vi "Dashboard Main.vi"() -> ()   [LabVIEW 2018]
uses:
  <vilib>/Utility/miscctls.llb/LVRowAndColumnTypeDef.ctl
  <vilib>/event_ctls.llb/eventvkey.ctl
  <vilib>/Rock Robotics/Network Tables/NT Read Numeric Array.vi
  <vilib>/Rock Robotics/WPI/Dashboard/WPI_DashboardLogging Global.vi
  <vilib>/Utility/inputDevices.llb/keyboardAcquire.vi
panel:
  out "keys pressed":T1(ring)=enum."RIGHT"
  in  "Camera Settings Right":T2={"Frame Rate"=30, "Compression"=30, "Size"=1, "DB Camera Config"=FALSE} {"Frame Rate" scale=1.0..30.0; "Compression" scale=100.0..-1.0; "Size" items=["640x480", "320x240", "160x120"]}
  in  "Camera Name Right":string(combo)="No Camera Selection"
  out "Camera Perf":string
  in  "Camera Settings":T2={"Frame Rate"=30, "Compression"=30, "Size"=1, "DB Camera Config"=FALSE} {"Frame Rate" scale=1.0..30.0; "Compression" scale=100.0..-1.0; "Size" items=["640x480", "320x240", "160x120"]}
  in  "TCP":refnum<k5>
  in  "Rec Mode":enum32{"Stop", "Record", "Playback"}(radio)
  out "Robot IP":string
  out "Image Message":string="Timeout in Camera Communications"
  in  "Dashboard Tab":T3(tab)
  out "tour hauteur":dbl(slide) caption="Slide 2" scale=0.0..500.0
  out "Encodeur tour":dbl(slide) caption="Slide" scale=0.0..500.0
  in  "Select Auto":string(combo)="Select Autonomous ..."
  out "NT Connection":bool
  out "MotorChart R":cluster{"Numeric":dbl, "Numeric":dbl}(graph)
  out "MotorChart L":cluster{"Numeric":dbl, "Numeric":dbl}(graph)
  out "MotorSliders R":cluster{"MotorSlide1":dbl, "MotorSlide2":dbl} {"MotorSlide2" scale=-1.0..1.0 scale format="%#_2e"; "MotorSlide1" scale=-1.0..1.0 scale format="%#_2e"}
  out "MotorSliders L":cluster{"MotorSlide1":dbl, "MotorSlide2":dbl} {"MotorSlide2" scale=-1.0..1.0 scale format="%#_2e"; "MotorSlide1" scale=-1.0..1.0 scale format="%#_2e"}
  out "JS1 Z":dbl(slide) scale=-1.0..1.0 scale format="%#_2e"
  out "JS1 Graph":cluster{"X":dbl, "Y":dbl}[](graph)
  out "JS1 Buttons":T4
  out "JS2 Z":dbl(slide) scale=-1.0..1.0 scale format="%#_2e"
  out "JS2 Graph":cluster{"X":dbl, "Y":dbl}[](graph)
  out "JS2 Buttons":T4
  out "Mode":T5(ring)=enum."Auto Disabled"
  out "Right Camera Perf":cluster{"Bandwidth (Mbps)":dbl, "FPS":dbl}
  out "Camera Image Right":T6(plugin-control)
  in  "DB/String 9":string
  in  "DB/String 8":string
  in  "DB/String 7":string
  in  "DB/String 6":string
  in  "DB/String 5":string
  in  "DB/String 4":string
  in  "DB/String 3":string
  in  "DB/String 2":string
  in  "DB/String 1":string
  in  "DB/String 0":string
  in  "DB/Slider 0":dbl(slide) scale=0.0..5.0
  in  "DB/Slider 1":dbl(slide) scale=0.0..5.0
  in  "DB/Slider 2":dbl(slide) scale=0.0..5.0
  in  "DB/Slider 3":dbl(slide) scale=0.0..5.0
  out "DB/LED 3":bool
  out "DB/LED 2":bool
  out "DB/LED 1":bool
  out "DB/LED 0":bool
  in  "DB/Button 3":bool
  in  "DB/Button 2":bool
  in  "DB/Button 1":bool
  in  "DB/Button 0":bool caption="New Name"
  in  "Test Slider":dbl(slide) scale=0.0..100.0 scale format="%#_3g"
  in  "On/Off":bool caption="Solenoid"
  in  "Test Name":u16(ring) items=["Select the test to run..."]
  in  "Test Tree":string(tree)
  in  "Motor":cluster{"Value":dbl, "Enable":bool} {"Value" scale=-1.0..1.0 scale format="%#_3g"}
  out "Progress":T7 {"Test Progress" scale=0.0..100.0}
  in  "Rev/Fwd":cluster{"Forward":bool, "Reverse":bool}
  in  "Test Ring":u16(ring) items=["Monochrome", "Color"]
  out "Cmd Status":string
  in  "Execute Command":bool
  in  "Command Params":string[][](table)
  in  "Command Selection":i32(listbox)
  in  "CheckList":i32(listbox)
  out "Tree":string(tree)
  out "Camera Image":T6(plugin-control)
  out "Background":bool
  in  "Camera Name":string(combo)="No Camera Selection"
  # "HW"
  # "HW"
  # "Joysticks"
  # "Drive Motors"
  # "Front"
  # "Right"
  # "Left"
  # "Back"
  # "This tab is a great place for autonomous settings and robot-specific values.\nPlace controls and indicators inside this tab and match name to\nDashboard Variables on robot. You can also delete this comment."
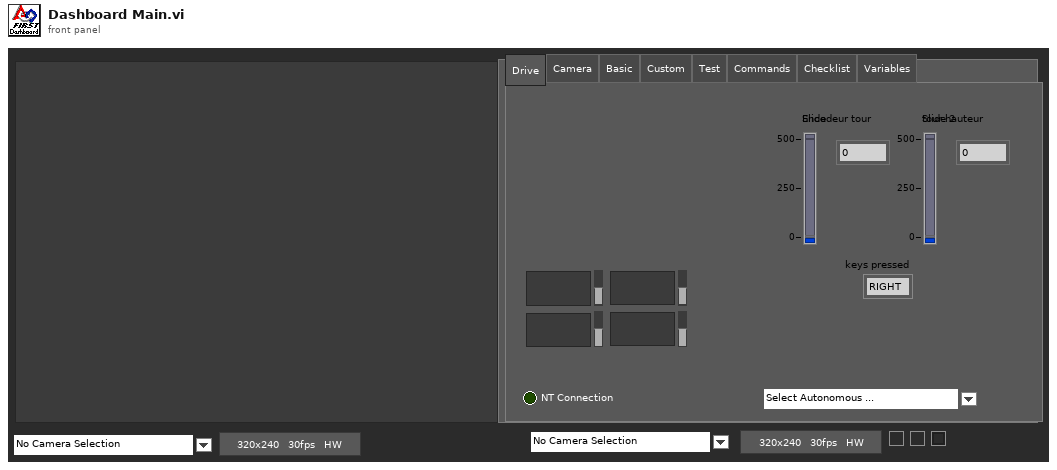
[diagram p1: front panel]
types:
  T1 = enum16{"0", "1", "2", "3", "4", "5", "6", "7", "8", "9", "A", "B", "C", "D", "E", "F", "G", "H", "I", "J", "K", "L", "M", "N", "O", "P", "Q", "R", "S", "T", "U", "V", "W", "X", "Y", "Z", "F1", "F2", "F3", "F4", "F5", "F6", "F7", "F8", "F9", "F10", "F11", "F12", "F13", "F14", "F15", "ADD", "BACK", "BACKSLASH", "CAPITAL", "COMMA", "DECIMAL", "DELETE", "DIVIDE", "DOWN", "END", "EQUALS", "ESCAPE", "GRAVE (`)", "HOME", "INSERT", "LBRACKET", "LCONTROL", "LEFT", "L ALT", "LSHIFT", "LWIN", "MINUS", "MULTIPLY", "NEXT", "NUMLOCK", "NUMPAD_0", "NUMPAD_1", "NUMPAD_2", "NUMPAD_3", "NUMPAD_4", "NUMPAD_5", "NUMPAD_6", "NUMPAD_7", "NUMPAD_8", "NUMPAD_9", "PAUSE", "PERIOD", "PRIOR (PG UP)", "RBRACKET", "RCONTROL", "RETURN", "RIGHT", "R ALT", "RSHIFT", "RWIN", "SCROLL", "SEMICOLON", "SLASH", "SPACE", "SUBTRACT", "TAB", "UP", "ENTER (num pad)", "' (quote)"}
  T2 = cluster{"Frame Rate":i32, "Compression":i32, "Size":u16, "DB Camera Config":bool}
  T3 = enum32{"Drive", "Camera", "Basic", "Custom", "Test", "Commands", "Checklist", "Variables"}
  T4 = cluster{bool, bool, bool, bool, bool, bool, bool, bool, bool, bool, bool, bool}
  T5 = enum8{"Tele-Op Disabled", "Tele-Op Enabled", "Auto Disabled", "Auto Enabled", "Test Disabled", "Test Enabled", "Disconnected", "No Code", "E-Stop"}
  T6 = typedef "IMAQ Image.ctl" = refnum<image>
  T7 = cluster{"Test Progress":u8, "Test Progress Text":string}
  T8 = cluster{"Save Path":path, "Interval (s)":dbl, "Keep":i32}
  T9 = typedef "Image Type" = u32
  T10 = cluster{"IDs":cluster{"RPC field ID":u16, "Unique ID":u16}, "String":string}
  T11 = cluster{"Error Strings":string, "Disable Counts":cluster{u16, u16}, "Rail Faults":cluster{u16, u16, u16}, "Robot IP":string, "DB Mode":u8, "Event Info":cluster{"Name":string, "Type":u8, "Number":u16, "Replay":u8}}
  T12 = cluster{"Storage":cluster{"Disk Free":u64, "RAM Block":u32, "RAM free":u32}, "CPU Utilization":cluster{"CPU % ISR":sgl, "CPU % Time Crit":sgl, "CPU % Timed Str":sgl, "CPU % High":sgl, "CPU % Above":sgl, "CPU % Normal":sgl, "CPU % Low":sgl}, "CAN":cluster{"% Bus Utilization":sgl, "Bus Off Cnt":u32, "TX_FIFO Full Cnt":u32, "Receive Error Cnt":u8, "Transmit Error Cnt":u8}, "HID":cluster{"HID Outputs":u32, "Rumble Low":u16, "Rumble High":u16}[]}
  T13 = cluster{"Status bits":cluster{"Test Mode":bool, "Autonomous":bool, "Enabled":bool, "Code Start":bool, "Brownout":bool, "Reserved 2":bool, "Reserved 3":bool, "E-Stop":bool}, "Code Trace":cluster{"Disabled":bool, "TeleOp":bool, "Auto":bool, "Test":bool}, "Controller Type":enum16{"unknown", "cRIO", "roboRio"}, "Code?":enum16{"unknown", "noCode", "code"}, "Battery V":dbl}
  T14 = cluster{"Control Bits":cluster{"TestMode":bool, "Autonomous":bool, "Enabled":bool, "FMS Present":bool, bool, bool, bool, "E-Stop":bool}, "Team Station ":u8, "Countdown":sgl, "Joystick Values":cluster{"Axes":dbl[], "Buttons":bool[], "POVs":i16[]}[]}
  T15 = cluster{"Axes":dbl[], "Buttons":bool[], "POVs":i16[]}[]
  T16 = cluster{"Axes":dbl[], "Buttons":bool[], "POVs":i16[]}
  T17 = cluster{"Buttons[0]":bool, "Buttons[1]":bool, "Buttons[2]":bool, "Buttons[3]":bool, "Buttons[4]":bool, "Buttons[5]":bool, "Buttons[6]":bool, "Buttons[7]":bool, "Buttons[8]":bool, "Buttons[9]":bool, "Buttons[10]":bool, "Buttons[11]":bool}
  T18 = cluster{"Camera Image":refnum<vi>, "Dashboard Tab":refnum<vi>, "Background":refnum<vi>, "Rec Mode":refnum<vi>, "Test Slider":refnum<vi>, "On/Off ":refnum<vi>, "Test Ring":refnum<vi>, "Rev/Fwd":refnum<vi>, "Test Name":refnum<vi>, "Motor":refnum<vi>, "Progress":refnum<vi>, "CheckList":refnum<vi>, "Tree":refnum<vi>, "Test Tree":refnum<vi>, "Command Params":refnum<vi>, "Command Selection":refnum<vi>, "Execute Command":refnum<vi>, "Cmd Status":refnum<vi>, "Camera Settings":refnum<vi>, "Camera Name":refnum<vi>, "Camera Perf":refnum<vi>, "Camera Settings Right":refnum<vi>, "Camera Name Right":refnum<vi>, "Camera Image Right":refnum<vi>}
  T19 = cluster{"Global Rectangle":i32[], "Contours":cluster{"Contour Type":u32, "ROI Type":u32, "Points":i32[]}[]}
  T20 = cluster{"Camera Name":string, string, "Saved DB Images Info":cluster{"Save Path":path, "Interval (s)":dbl, "Keep":i32}}
  T21 = cluster{"Camera Name Right":string, string, "Saved DB Images Info":cluster{"Save Path":path, "Interval (s)":dbl, "Keep":i32}}
  T22 = enum16{"0", "1", "2", "3", "4", "5", "6", "7", "8", "9", "A", "B", "C", "D", "E", "F", "G", "H", "I", "J", "K", "L", "M", "N", "O", "P", "Q", "R", "S", "T", "U", "V", "W", "X", "Y", "Z", "F1", "F2", "F3", "F4", "F5", "F6", "F7", "F8", "F9", "F10", "F11", "F12", "F13", "F14", "F15", "ADD", "BACK", "BACKSLASH", "CAPITAL", "COMMA", "DECIMAL", "DELETE", "DIVIDE", "DOWN", "END", "EQUALS", "ESCAPE", "GRAVE (`)", "HOME", "INSERT", "LBRACKET", "LCONTROL", "LEFT", "L ALT", "LSHIFT", "LWIN", "MINUS", "MULTIPLY", "NEXT", "NUMLOCK", "NUMPAD_0", "NUMPAD_1", "NUMPAD_2", "NUMPAD_3", "NUMPAD_4", "NUMPAD_5", "NUMPAD_6", "NUMPAD_7", "NUMPAD_8", "NUMPAD_9", "PAUSE", "PERIOD", "PRIOR (PG UP)", "RBRACKET", "RCONTROL", "RETURN", "RIGHT", "R ALT", "RSHIFT", "RWIN", "SCROLL", "SEMICOLON", "SLASH", "SPACE", "SUBTRACT", "TAB", "UP", "ENTER (num pad)", "' (quote)"}[]
  T23 = cluster{"Operation":enum16{"Update", "Clear"}, "Color Box":u32}[]
  T24 = typedef "eventvkey.ctl" = enum16{"ASCII", "Enter", "Return", "Shift", "Ctrl", "Alt", "Cmd", "Opt", "Caps", "NumLock", "Clear", "Break", "Up", "Down", "Left", "Right", "Insert", "Delete", "Home", "End", "PageUp", "PageDown", "Escape", "Help", "Pause", "ScrollLock", "F1", "F2", "F3", "F4", "F5", "F6", "F7", "F8", "F9", "F10", "F11", "F12", "F13", "F14", "F15", "F16", "F17", "F18", "F19", "F20", "F21", "F22", "F23", "F24", "Play", "VolumeUp", "VolumeDown", "Mute", "Two Byte Char"}
  T25 = cluster{"Image Size":bool, "Image Type":bool, "Pixel Value":bool, "ROI Information":bool, "Zoom Factor":bool}
  T26 = cluster{"Operation":enum16{"Update", "Clear"}, "Color Box":u32}
  T27 = typedef "LVRowAndColumnTypeDef.ctl" = cluster{"Row":i32, "Column":i32}
  T28 = cluster{"Shift":bool, "Ctrl":bool, "Alt":bool, "Cmd":bool, "Opt":bool}
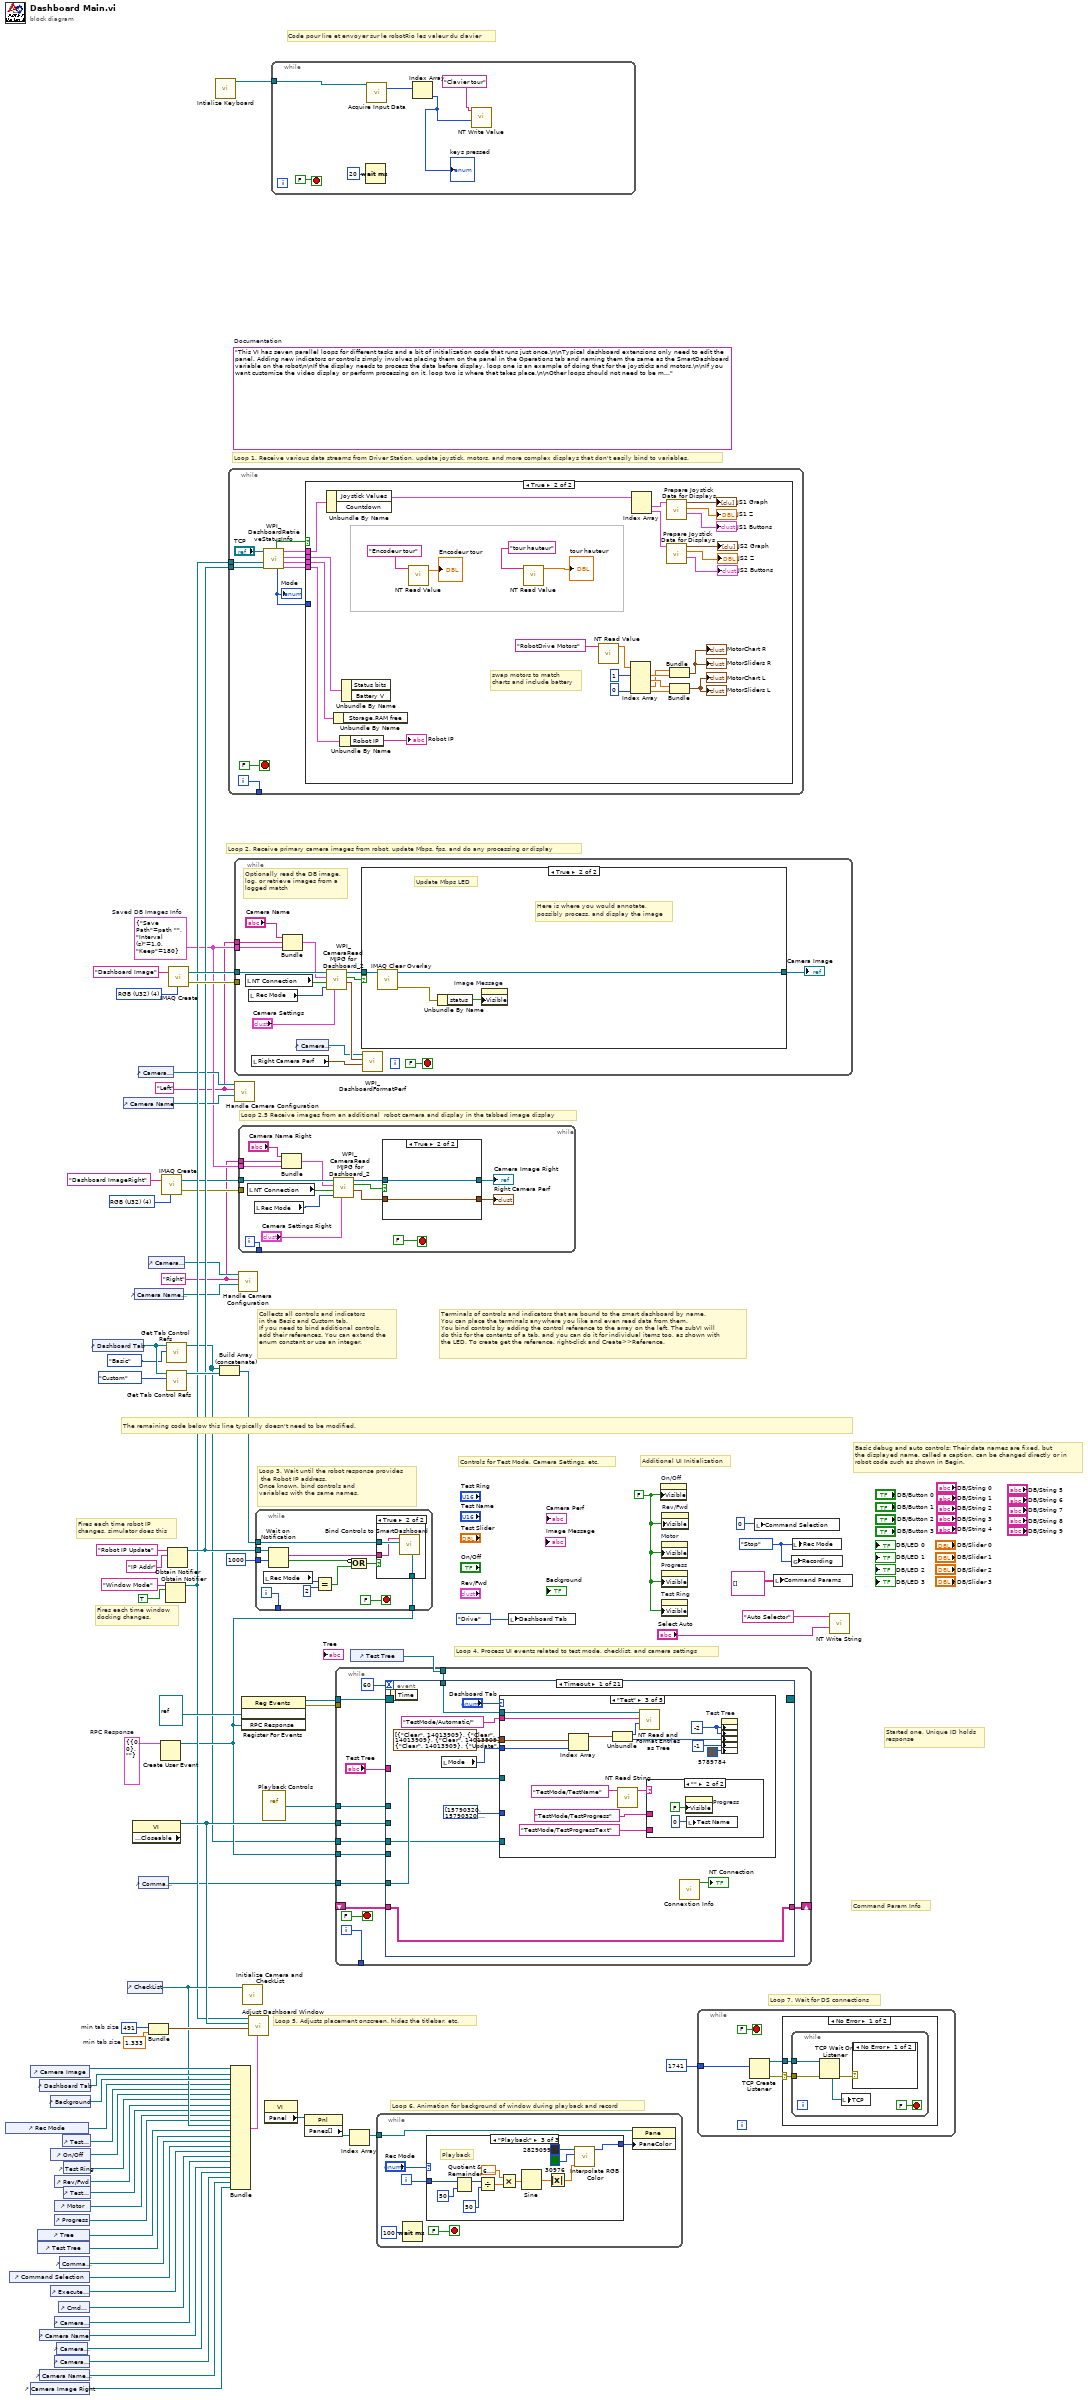
[diagram p0: block diagram]
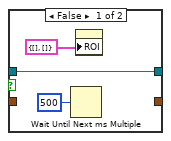
[diagram p2: hidden frame]
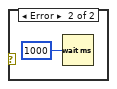
[diagram p3: hidden frame]
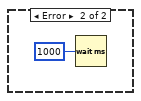
[diagram p4: hidden frame]
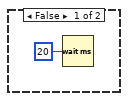
[diagram p5: hidden frame]
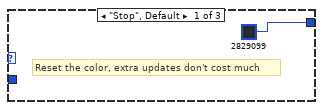
[diagram p6: hidden frame]
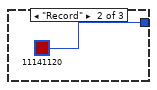
[diagram p7: hidden frame]
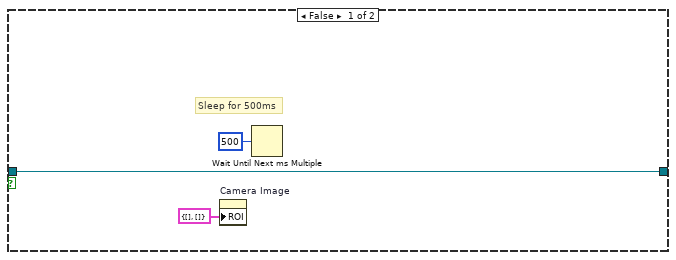
[diagram p9: hidden frame]
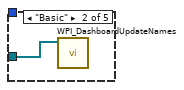
[diagram p11: hidden frame]
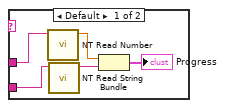
[diagram p12: hidden frame]
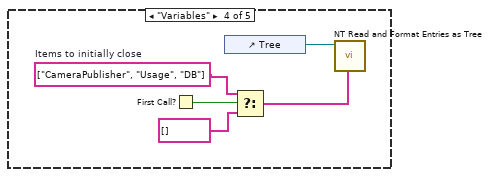
[diagram p13: hidden frame]
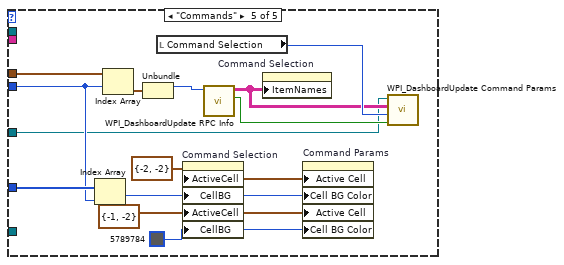
[diagram p14: hidden frame]
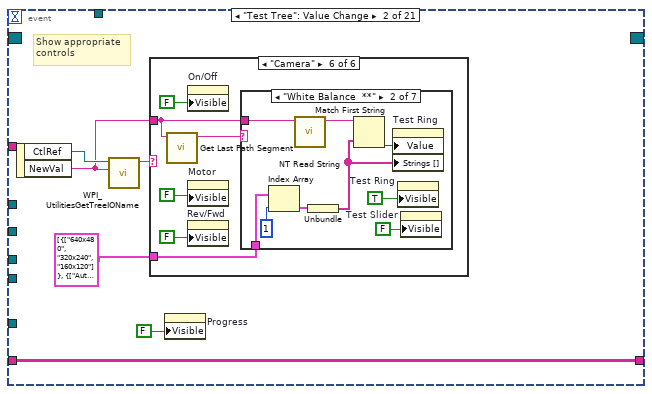
[diagram p15: hidden frame]
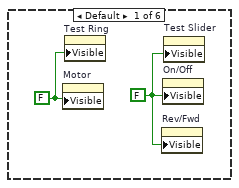
[diagram p16: hidden frame]
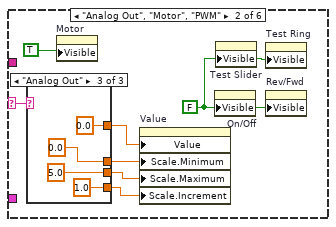
[diagram p17: hidden frame]
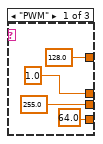
[diagram p18: hidden frame]
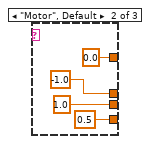
[diagram p19: hidden frame]
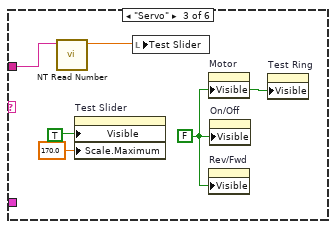
[diagram p20: hidden frame]
diagram:
  w4 = T8 {"Save Path"=path "", "Interval (s)"=1.0, "Keep"=180}  # Saved DB Images Info
  w3 = "Right"
  w2 = "Left"
  w14 = T9 4 items=["Grayscale (U8)", "Grayscale (I16)", "Grayscale (SGL)", "Complex (CSG)", "RGB (U32)", "HSL (U32)", "RGB (U64)"] ("Image Type")
  w30 = T10 {"IDs"={"RPC field ID"=0, "Unique ID"=0}, "String"=""}  # RPC Response
  w53 = 491  # min tab size
  w52 = 1.333  # min tab size
  w60 = enum32{"Stop", "Record", "Playback"}."Stop" ("Rec Mode")
  w37 = FALSE ("Visible")
  (unwired) "This VI has seven parallel loops for different tasks and a bit of initialization code that runs just once.\n\nTypical dashboard extensions only need to edit the panel. Adding new indicators or controls simply involves placing them on the panel in the Operations tab and naming them the same as the SmartDashboard variable on the robot\n\nIf the display needs to process the data before display, loop one is an example of doing that for the joysticks and motors.\n\nIf you want customize the video display or perform processing on it, loop two is where that takes place.\n\nOther loops should not need to be modified. They are pretty standard, and document the task they perform."  # Documentation
  w77 = T9 4 items=["Grayscale (U8)", "Grayscale (I16)", "Grayscale (SGL)", "Complex (CSG)", "RGB (U32)", "HSL (U32)", "RGB (U64)"] ("Image Type")
  # "Code pour lire et envoyer sur le robotRio les valeur du clavier"
  # "Loop 2.5 Receive images from an additional  robot camera and display in the tabbed image display"
  # "Command Param Info"
  # "Started one, Unique ID holds\nresponse"
  # "Loop 7. Wait for DS connections"
  # "Basic debug and auto controls: Their data names are fixed, but\nthe displayed name, called a caption, can be changed directly or in\nrobot code such as shown in Begin."
  # "Controls for Test Mode, Camera Settings, etc."
  # "Additional UI Initialization"
  # "Loop 6. Animation for background of window during playback and record"
  # "Fires each time robot IP\nchanges, simulator does this"
  # "Fires each time window\ndocking changes."
  # "Collects all controls and indicators\nin the Basic and Custom tab.\nIf you need to bind additional controls,\nadd their references. You can extend the\nenum constant or use an integer."
  # "The remaining code below this line typically doesn't need to be modified."
  # "Loop 4. Process UI events related to test mode, checklist, and camera settings"
  # "Terminals of controls and indicators that are bound to the smart dashboard by name.\nYou can place the terminals anywhere you like and even read data from them.\nYou bind controls by adding the control reference to the array on the left. The subVI will\ndo this for the contents of a tab, and you can do it for individual items too, as shown with\nthe LED. To create get the reference, right-click and Create>>Reference."
  # "Loop 3. Wait until the robot response provides\n the Robot IP address.\nOnce known, bind controls and\nvariables with the same names."
  # "Loop 5. Adjusts placement onscreen, hides the titlebar, etc."
  # "Loop 1. Receive various data streams from Driver Station, update joystick, motors, and more complex displays that don't easily bind to variables."
  # "Loop 2. Receive primary camera images from robot, update Mbps, fps, and do any processing or display"
  n1 = control-ref of="Rec Mode"() -> (w43:refnum<vi>)
  n2 = control-ref of="Command Selection"() -> (w29:refnum<vi>)
  n3 = control-ref of="Camera Image Right"() -> (w7:refnum<vi>)
  n4 = control-ref of="Camera Image"() -> (w55:refnum<vi>)
  n5 = control-ref of="Tree"() -> (w47:refnum<vi>)
  n6 = control-ref of="Test Tree"() -> (w46:refnum<vi>)
  n7 = control-ref of="Dashboard Tab"() -> (w54:refnum<vi>)
  n8 = control-ref of="Camera Name"() -> (w20:refnum<vi>)
  n9 = control-ref of="Camera Name Right"() -> (w8:refnum<vi>)
  n10 = control-ref of="Execute Command"() -> (w31:refnum<vi>)
  n11 = control-ref of="Background"() -> (w50:refnum<vi>)
  n12 = control-ref of="On/Off"() -> (w41:refnum<vi>)
  n13 = control-ref of="Progress"() -> (w38:refnum<vi>)
  n14 = control-ref of="Camera Settings"() -> (w21:refnum<vi>)
  n15 = control-ref of="Camera Settings Right"() -> (w9:refnum<vi>)
  n16 = control-ref of="Rev/Fwd"() -> (w39:refnum<vi>)
  n17 = control-ref of="Motor"() -> (w44:refnum<vi>)
  n18 = control-ref of="Camera Perf"() -> (w19:refnum<vi>)
  n19 = control-ref of="Cmd Status"() -> (w25:refnum<vi>)
  n20 = control-ref of="Command Params"() -> (w32:refnum<vi>)
  n21 = control-ref of="Test Slider"() -> (w42:refnum<vi>)
  n22 = control-ref of="Test Ring"() -> (w40:refnum<vi>)
  n23 = control-ref of="Test Name"() -> (w45:refnum<vi>)
  n24 = control-ref of="Dashboard Tab"() -> (w58:refnum<vi>)
  n25 = control-ref of="Camera Name"() -> (w22:refnum<vi>)
  n26 = control-ref of="CheckList"() -> (w48:refnum<vi>)
  n27 = property class="VI" props=["Front Panel.Closeable"]() -> (reference out=w59:refnum<vi>)  [unwired: 2 in, 2 out]
  n28 = control-ref of="Camera Name Right"() -> (w10:refnum<vi>)
  n29 = control-ref of="Camera Settings"() -> (w23:refnum<vi>)
  n30 = control-ref of="Command Params"() -> (w24:refnum<vi>)
  n31 = control-ref of="Camera Settings Right"() -> (w11:refnum<vi>)
  n32 = Bundle("min tab size"=w53, "min tab size"=w52) -> (w51:cluster{"min tab size":i32, "min tab size":dbl})  [unwired: 1 in]
  n33 = Create User Event(user event datatype=w30) -> (user event=w26:refnum<user-event>)  [unwired: 1 in, 1 out]
  n34 = call "IMAQ Create"("Image Name"="Dashboard ImageRight", "Image Type"=w14) -> ("New Image"=w13:T6, "error out"=w12:errorcluster)  [unwired: 2 in, 1 out]
  n35 = Obtain Notifier(name (unnamed)="Window Mode", notification data type=TRUE) -> (notifier out=w35:refnum<notifier>)  [unwired: 2 in, 2 out]
  n36 = call <vilib>:"Get Tab Control Refs.vi"("Page Index"=T3."Basic" ("Dashboard Tab"), "TabControl in"=w58) -> ("ControlsOnPage"=w18:refnum<vi>[])  [unwired: 9 in]
  n37 = call <vilib>:"Get Tab Control Refs.vi"("Page Index"=T3."Custom" ("Dashboard Tab"), "TabControl in"=w58) -> ("ControlsOnPage"=w57:refnum<vi>[])  [unwired: 9 in]
  n38 = Obtain Notifier(name (unnamed)="Robot IP Update", notification data type="IP Addr" ("name (unnamed)")) -> (notifier out=w36:refnum<notifier>)  [unwired: 2 in, 2 out]
  n39 = call "IMAQ Create"("Image Name"="Dashboard Image", "Image Type"=w77) -> ("New Image"=w75:T6, "error out"=w74:errorcluster)  [unwired: 2 in, 1 out]
  n40 = call <vilib>:"Intialize Keyboard.vi"() -> ("device ID"=w1:refnum<k1>)  [unwired: 10 in, 1 out]
  n41 = Build Array (concatenate)(w18, w57) -> (w56:refnum<vi>[])
  n42 = while {
    tunnel: [w87] -> _
    tunnel: w36 -> [w81]
    tunnel: w35 -> [w78]
    i -> [w87]
    stop <- FALSE stop-if-true
    n43 = call <vilib>:"WPI_DashboardRetrieveStatusInfo.vi"("Binding Refnum"=w81, "Window Mode Notifier"=w78, "TCP Cnx"="TCP") -> ("Power and Errors"=w82:T11, "Robot Metrics"=w85:T12, "Status Info"=w86:T13, "Control Info"=w83:T14, "Robot Mode"=w80:T5, "Process?"=w84:bool)  [unwired: 3 in]
    "Mode" <- w80
    n44 = case shown="True" w84 {
      tunnel: w86 -> [_ w117]
      tunnel: w85 -> [_ w116]
      tunnel: w83 -> [_ w115]
      tunnel: w82 -> [_ w114]
      tunnel: w80 -> [_ _]
      frame False {
        n45 = Wait (ms)(milliseconds to wait=u32 20) -> ()  [unwired: 1 out]
      }
      frame True {
        # "swap motors to match\ncharts and include battery"
        n46 = Unbundle By Name(w115) -> ("Joystick Values"=w105:T15)  [unwired: 1 out]
        n47 = Unbundle By Name(w116) -> ()  [unwired: 1 out]
        n48 = Unbundle By Name(w114) -> ("Robot IP"=→"Robot IP":string)
        n49 = Unbundle By Name(w117) -> ()  [unwired: 2 out]
        n50 = call-poly <vilib>:"NT Read Value.vi"("Name"="Encodeur tour") -> ("Numeric"=→"Encodeur tour":dbl)  [unwired: 9 in, 1 out]
        n51 = call-poly <vilib>:"NT Read Value.vi"("Name"="tour hauteur") -> ("Numeric"=→"tour hauteur":dbl)  [unwired: 9 in, 1 out]
        n52 = call-poly <vilib>:"NT Read Value.vi"("Name"="RobotDrive Motors") -> ("Numeric Array"=w95:dbl[])  [unwired: 9 in, 1 out]
        n53 = Index Array(array=w95, index #1=1, index #4=0) -> (element #1=w109:dbl, element #2=w110:dbl, element #3=w108:dbl, element #4=w113:dbl)  [unwired: 2 in]
        n54 = Index Array(array=w105) -> (element #1=w104:T16, element #2=w100:T16)  [unwired: 2 in]
        n55 = call "Prepare Joystick Data for Displays.vi"("Joystick Values"=w100) -> ("Buttons"=→"JS2 Buttons":T17, "Z Axis"=→"JS2 Z":dbl, "Cartesian Data"=→"JS2 Graph":cluster{"X axis":dbl, "X axis":dbl}[])  [unwired: 8 in]
        n56 = call "Prepare Joystick Data for Displays.vi"("Joystick Values"=w104) -> ("Buttons"=→"JS1 Buttons":T17, "Z Axis"=→"JS1 Z":dbl, "Cartesian Data"=→"JS1 Graph":cluster{"X axis":dbl, "X axis":dbl}[])  [unwired: 8 in]
        n57 = Bundle("Numeric"=w108, "Numeric"=w109) -> (→"MotorChart R" →"MotorSliders R":cluster{"Numeric":dbl, "Numeric":dbl})  [unwired: 1 in]
        n58 = Bundle("Numeric"=w110, "Numeric"=w113) -> (→"MotorChart L" →"MotorSliders L":cluster{"Numeric":dbl, "Numeric":dbl})  [unwired: 1 in]
      }
    }
  }
  n59 = Bundle("Camera Image"=w55, "Dashboard Tab"=w54, "Background"=w50, "Rec Mode"=w43, "Test Slider"=w42, "On/Off"=w41, "Test Ring"=w40, "Rev/Fwd"=w39, "Test Name"=w45, "Motor"=w44, "Progress"=w38, "CheckList"=w48, "Tree"=w47, "Test Tree"=w46, "Command Params"=w32, "Command Selection"=w29, "Execute Command"=w31, "Cmd Status"=w25, "Camera Settings"=w21, "Camera Name"=w20, "Camera Perf"=w19, "Camera Settings Right"=w9, "Camera Name Right"=w8, "Camera Image Right"=w7) -> (w49:T18)  [unwired: 1 in]
  n60 = call "Handle Camera Configuration.vi"("CameraNameRef"=w22, "Display Name"=w2, "ClusterRef"=w23) -> ()  [unwired: 9 in]
  n61 = while {
    tunnel: w75 -> [w131]
    tunnel: w74 -> [_]
    tunnel: w4 -> [w124]
    tunnel: w2 -> [w121]
    stop <- FALSE stop-if-true
    # "Optionally read the DB image,\nlog, or retrieve images from a\nlogged match"
    n62 = local read "NT Connection"() -> (w125:bool)
    n63 = local read "Rec Mode"() -> (w128:enum32{"Stop", "Record", "Playback"})
    n64 = local read "Right Camera Perf"() -> (w119:cluster{"Bandwidth (Mbps)":dbl, "FPS":dbl})
    n65 = Bundle("Camera Name"="Camera Name", w121, "Saved DB Images Info"=w124) -> (w123:T20)  [unwired: 1 in]
    n66 = control-ref of="Camera Perf"() -> (w118:refnum<vi>)
    n67 = call <vilib>:"WPI_CameraRead MJPG for Dashboard_2.vi"("Camera Settings"="Camera Settings", "Rec Mode"=w128, "NT Connection"=w125, "Capture Info"=w123, "Image in"=w131) -> ("perf info"=w120:cluster{"Bandwidth (Mbps)":dbl, "fps":dbl}, "Active"=w129:bool, "Image\\ out"=w130:T6)  [unwired: 4 in]
    n68 = case shown="True" w129 {
      tunnel: w130 -> [w134 w137]
      tunnel: [w134 w136] -> w126
      frame False {
        # "Sleep for 500ms"
        n69 = property on="Camera Image" class="ImageControl"("ROI"=T19 {"Global Rectangle"=[], "Contours"=[]}) -> ()  [unwired: 2 in, 2 out]
        n70 = Wait Until Next ms Multiple(millisecond multiple=u32 500) -> ()  [unwired: 1 out]
      }
      frame True {
        # "Here is where you would annotate,\npossibly process, and display the image"
        # "Update Mbps LED"
        n71 = call "IMAQ Clear Overlay"("Image"=w137) -> ("error out"=w138:errorcluster, "Image Out"=w136:T6)  [unwired: 2 in, 7 out]
        n72 = Unbundle By Name(w138) -> ("status"=w139:bool)
        n73 = property on="Image Message" class="Str"("Visible"=w139) -> ()  [unwired: 2 in, 2 out]
      }
    }
    "Camera Image" <- w126
    n74 = call <vilib>:"WPI_DashboardFormatPerf.vi"("Right Camera Perf"=w119, "Performance"=w120, "String in"=w118) -> ()  [unwired: 9 in]
  }
  n75 = call "Handle Camera Configuration.vi"("CameraNameRef"=w10, "Display Name"=w3, "ClusterRef"=w11) -> ()  [unwired: 9 in]
  n76 = while {
    tunnel: w13 -> [w154]
    tunnel: w12 -> [_]
    tunnel: [w149] -> _
    tunnel: w4 -> [w145]
    tunnel: w3 -> [w142]
    i -> [w149]
    stop <- FALSE stop-if-true
    n77 = local read "NT Connection"() -> (w146:bool)
    n78 = local read "Rec Mode"() -> (w153:enum32{"Stop", "Record", "Playback"})
    n79 = Bundle("Camera Name Right"="Camera Name Right", w142, "Saved DB Images Info"=w145) -> (w144:T21)  [unwired: 1 in]
    n80 = call <vilib>:"WPI_CameraRead MJPG for Dashboard_2.vi"("Camera Settings"="Camera Settings Right", "Rec Mode"=w153, "NT Connection"=w146, "Capture Info"=w144, "Image in"=w154) -> ("perf info"=w140:cluster{"Bandwidth (Mbps)":dbl, "fps":dbl}, "Active"=w148:bool, "Image\\ out"=w151:T6)  [unwired: 4 in]
    n81 = case shown="True" w148 {
      tunnel: w151 -> [w156 w159]
      tunnel: [w156 w159] -> w147
      tunnel: [_ w158] -> w141
      tunnel: w140 -> [_ w158]
      frame False {
        n82 = Wait Until Next ms Multiple(millisecond multiple=u32 500) -> ()  [unwired: 1 out]
        n83 = property on="Camera Image Right" class="ImageControl"("ROI"=T19 {"Global Rectangle"=[], "Contours"=[]}) -> ()  [unwired: 2 in, 2 out]
      }
      frame True {
      }
    }
    "Camera Image Right" <- w147
    "Right Camera Perf" <- w141
  }
  n84 = register-events(refnum<vi> refnum, w26) -> (reference out=w64:refnum<event-registration>, error out=w63:errorcluster)  [unwired: 2 in]
  n85 = call "Initialize Camera and CheckList.vi"("ListBox in"=w48) -> ()  [unwired: 11 in]
  n86 = call "Adjust Dashboard Window.vi"("Sizing Refnums"=w49, "Size Constraints"=w51, "VI"=w59, "WIn Mode"=w35) -> ()  [unwired: 8 in]
  n87 = while {
    tunnel: w56 -> [w171]
    tunnel: w36 -> [w169]
    tunnel: [w167] -> _
    tunnel: u32 1000 ("milliseconds to wait") -> [w166]
    tunnel: w26 -> [w160]
    i -> [w167]
    stop <- FALSE stop-if-true
    n88 = local read "Rec Mode"() -> (w162:enum32{"Stop", "Record", "Playback"})
    n89 = Wait on Notification(notifier=w169, timeout in ms (-1)=w166) -> (notification=w168:string, timed out?=w164:bool)  [unwired: 2 in, 2 out]
    n90 = Equal?(x=w162, y=u16 2 ("Rec Mode")) -> (x = y?=w163:bool)
    n91 = Compound Arithmetic op=OR(invert w164, w163) -> (w165:bool)
    n92 = case shown="True" w165 {
      tunnel: w171 -> [_ w174]
      tunnel: w168 -> [_ w173]
      tunnel: w160 -> [_ w172]
      frame False {
      }
      frame True {
        n93 = call <vilib>:"Bind Controls to SmartDashboard.vi"("RPC ref"=w172, "Bound Control Refs"=w174, "Server IP Address"=w173) -> ()  [unwired: 9 in]
      }
    }
  }
  n94 = vi-ref "Playback Controls.vi"() -> (w65:refnum<vi>)
  n95 = property class="VI"() -> ("Panel"=w67:refnum<vi>)  [unwired: 2 in, 2 out]
  n96 = while {
    tunnel: w1 -> [w179]
    stop <- FALSE stop-if-true
    n97 = Wait (ms)(milliseconds to wait=u32 20) -> ()  [unwired: 1 out]
    n98 = call-poly <vilib>:"Acquire Input Data.vi"("device ID"=w179) -> ("keys pressed"=w177:T22)  [unwired: 16 in, 2 out]
    n99 = Index Array(array=w177) -> (element=w175:T1)  [unwired: 1 in]
    "keys pressed" <- w175
    n100 = call-poly <vilib>:"NT Write Value.vi"("Numeric"=w175, "Name"="Clavier tour") -> ()  [unwired: 9 in, 1 out]
  }
  n101 = property class="Pnl"(reference=w67) -> ("Panes[]"=w68:refnum<vi>[])  [unwired: 1 in, 2 out]
  n102 = Index Array(array=w68) -> (element=w66:refnum<vi>)  [unwired: 1 in]
  n103 = control-ref of="Test Tree"() -> (w69:refnum<vi>)
  n104 = while {
    tunnel: [w190] -> _
    tunnel: w69 -> [w189]
    tunnel: w65 -> [w188]
    tunnel: w64 -> [w187]
    tunnel: w63 -> [_]
    tunnel: w59 -> [w186]
    tunnel: w26 -> [w185]
    tunnel: w24 -> [w184]
    shift-right: [w183] -> _
    shift-left: _ -> [w182]
    tunnel: w18 -> [w181]
    i -> [w190]
    stop <- FALSE stop-if-true
    n105 = event shown="[0] Timeout" {
      selector: w187 -> [_ _ _ _ _ _ _ _ _ _ _ _ _ _ _ _ _ _ _ _ _]
      dyn-events: [_ _ _ _ _ _ _ _ _ _ _ _ _ _ _ _ w450 _ _ _ _] -> _
      timeout: u32 60 ("milliseconds to wait") -> [_ _ _ _ _ _ _ _ _ _ _ _ _ _ _ _ _ _ _ _ _]
      tunnel: w189 -> [w202 _ _ _ _ _ _ _ _ _ _ _ _ _ _ _ _ _ _ _ _]
      tunnel: "Test Tree" -> [_ _ _ _ _ _ _ _ _ _ _ w417 w425 w427 w431 w439 _ _ _ _ _]
      tunnel: w188 -> [_ _ _ _ _ _ _ _ _ _ _ _ _ _ _ _ w452 _ w470 _ _]
      tunnel: w186 -> [_ _ _ _ _ _ _ _ _ _ _ _ _ _ _ _ w448 _ _ _ _]
      tunnel: w185 -> [_ _ _ _ _ _ _ _ _ _ _ _ _ _ _ _ w446 _ _ _ _]
      tunnel: w184 -> [w197 _ _ _ _ _ w368 _ _ _ _ _ _ _ _ _ _ _ _ _ _]
      tunnel: [w196 w245 w347 w352 w361 w365 w366 w375 w385 w392 w404 w416 w423 w426 w430 w438 w445 w465 w467 w471 w484] -> w183
      tunnel: w182 -> [w196 w245 w347 w352 w361 w365 w366 _ _ w392 w404 w416 w423 w426 w430 w438 w445 w465 w467 w471 w484]
      tunnel: w181 -> [w194 _ _ _ _ _ _ _ _ _ _ _ _ _ _ _ _ _ _ _ _]
      event Timeout {
        n106 = event-data() -> ()  [unwired: 1 in, 1 out]
        n107 = local read "Mode"() -> (w199:T5)
        n108 = case shown="\"Test\"" "Dashboard Tab" {
          tunnel: w202 -> [_ _ w218 _ _]
          tunnel: "TestMode/Automatic/" ("Name Pattern") -> [_ _ w217 _ _]
          tunnel: T23 [{"Operation"=enum."Clear", "Color Box"=14013909}, {"Operation"=enum."Clear", "Color Box"=14013909}, {"Operation"=enum."Clear", "Color Box"=14013909}, {"Operation"=enum."Clear", "Color Box"=14013909}, {"Operation"=enum."Update", "Color Box"=14013909}, {"Operation"=enum."Update", "Color Box"=16777215}, {"Operation"=enum."Clear", "Color Box"=14013909}, {"Operation"=enum."Clear", "Color Box"=14013909}, {"Operation"=enum."Clear", "Color Box"=14013909}] -> [_ _ w210 _ w238]
          tunnel: w199 -> [_ _ w209 _ w237]
          tunnel: u32[] [15790320, 15790320, 15790320, 15790320, 16777215, 16777215, 15790320, 15790320, 15790320] -> [_ _ _ _ w243]
          tunnel: w197 -> [_ _ _ _ w231]
          tunnel: w194 -> [_ w204 _ _ _]
          frame "Custom", Default {
          }
          frame "Basic" {
            n109 = call <vilib>:"WPI_DashboardUpdateNames.vi"("Controls on Tab"=w204) -> ()  [unwired: 11 in]
          }
          frame "Test" {
            w216 = -2 ("Active Item:Row Number")
            n110 = Index Array(array=w210, index=w209) -> (element=w211:T26)
            n111 = Unbundle(w211) -> ("Operation"=w212:enum16{"Update", "Clear"}, "Color Box"=w213:u32)
            n112 = call <vilib>:"NT Read String.vi"("Name"="TestMode/TestName") -> ("String"=w207:string)  [unwired: 9 in, 1 out]
            n113 = call <vilib>:"NT Read and Format Entries as Tree.vi"("Operation"=w212, "Name Pattern"=w217, "Tree Refnum"=w218) -> ()  [unwired: 7 in, 2 out]
            n114 = case shown="\"\"" w207 {
              tunnel: "TestMode/TestProgress" ("Name") -> [w220 _]
              tunnel: "TestMode/TestProgressText" ("Name") -> [w219 _]
              frame Default {
                n115 = call <vilib>:"NT Read Number.vi"("Name"=w220) -> ("Numeric"=w221:dbl)  [unwired: 9 in, 1 out]
                n116 = call <vilib>:"NT Read String.vi"("Name"=w219) -> ("String"=w222:string)  [unwired: 9 in, 1 out]
                n117 = Bundle("Numeric"=w221, "String"=w222) -> (→"Progress":cluster{"Numeric":dbl, "String":string})  [unwired: 1 in]
              }
              frame "" {
                n118 = property on="Progress" class="Clust (strict)"("Visible"=FALSE) -> ()  [unwired: 2 in, 2 out]
                n119 = local write "Test Name"(u16 0) -> ()
              }
            }
            n120 = property on="Test Tree" class="Tree (strict)"("Active Item Row Number"=w216, "ActiveColNum"=w216, "CellBG"=w213, "Active Item Row Number"=-1 ("Active Item:Row Number"), "CellBG"=u32 5789784 ("Color Box")) -> ()  [unwired: 2 in, 2 out]
          }
          frame "Variables" {
            w228 = string[] ["CameraPublisher", "Usage", "DB"]  # Items to initially close
            n121 = First Call?() -> (First Call?: T/F=w229:bool)
            n122 = control-ref of="Tree"() -> (w230:refnum<vi>)
            n123 = Select(t=w228, s=w229, f=string[] []) -> (s? t:f=w226:string[])
            n124 = call <vilib>:"NT Read and Format Entries as Tree.vi"("Tags to  Close"=w226, "Tree Refnum"=w230) -> ()  [unwired: 8 in, 2 out]
          }
          frame "Commands" {
            w239 = u32 5789784 ("Color Box")
            w240 = T27 {"Row"=-1, "Column"=-2} ("Active Cell:Active Cell")
            w242 = T27 {"Row"=-2, "Column"=-2} ("Active Cell:Active Cell")
            n125 = Index Array(array=w243, index=w237) -> (element=w241:u32)
            n126 = Index Array(array=w238, index=w237) -> (element=w236:T26)
            n127 = Unbundle(w236) -> ("Operation"=w235:enum16{"Update", "Clear"})  [unwired: 1 out]
            n128 = local read "Command Selection"() -> (w234:i32)
            n129 = property on="Command Selection" class="MCListbox (strict)"("ActiveCell"=w242, "CellBG"=w241, "ActiveCell"=w240, "CellBG"=w239) -> ()  [unwired: 2 in, 2 out]
            n130 = call <vilib>:"WPI_DashboardUpdate RPC Info.vi"("Operation"=w235) -> ("update"=w233:bool, "commands"=w232:string[][])  [unwired: 9 in]
            n131 = property on="Command Selection" class="MCListbox (strict)"("ItemNames"=w232) -> ()  [unwired: 2 in, 2 out]
            n132 = property on="Command Params" class="Tbl (strict)"("Active Cell"=w242, "Cell BG Color"=w241, "Active Cell"=w240, "Cell BG Color"=w239) -> ()  [unwired: 2 in, 2 out]
            n133 = call <vilib>:"WPI_DashboardUpdate Command Params.vi"("Update"=w233, "NewVal"=w234, "Commands"=w232, "Param Tbl"=w231) -> ()  [unwired: 7 in, 1 out]
          }
        }
        n134 = call <vilib>:"Connextion Info.vi"() -> ("Connected"=→"NT Connection":bool)  [unwired: 10 in, 1 out]
      }
      event "Test Tree": Value Change {
        # "Show appropriate\ncontrols"
        n135 = event-data() -> ("CtlRef"=w248:refnum<vi>, "NewVal"=w246:string)  [unwired: 1 in]
        n136 = call <vilib>:"WPI_UtilitiesGetTreeIOName.vi"("NewVal"=w246, "TreeControl in"=w248) -> ("I/O Name"=w249:string)  [unwired: 9 in]
        n137 = case shown="\"Camera\"" w249 {
          selector: w249 -> [_ w256 _ w278 w287 _]
          tunnel: w246 -> [_ _ w275 w277 _ w294]
          tunnel: cluster{string[]}[] [{["640x480", "320x240", "160x120"]}, {["Auto", "Fixed indoor", "Fixed outdoor 1", "Fixed outdoor 2", "Fixed fluorescent 1", "Fixed fluorescent 2", "Hold current"]}, {["Auto", "Flicker-free 50 Hz", "Flicker-free 60 Hz", "Hold current"]}, {["None", "Prioritize frame rate", "Prioritize image quality"]}, {["Monochrome", "Color"]}] -> [_ _ _ _ _ w293]
          frame Default {
            w251 = FALSE ("Visible")
            w250 = FALSE ("Visible")
            n138 = property on="Motor" class="Clust (strict)"("Visible"=w250) -> ()  [unwired: 2 in, 2 out]
            n139 = property on="Test Ring" class="Ring (strict)"("Visible"=w250) -> ()  [unwired: 2 in, 2 out]
            n140 = property on="Rev/Fwd" class="Clust (strict)"("Visible"=w251) -> ()  [unwired: 2 in, 2 out]
            n141 = property on="On/Off" class="Bool (strict)"("Visible"=w251) -> ()  [unwired: 2 in, 2 out]
            n142 = property on="Test Slider" class="Slide (strict)"("Visible"=w251) -> ()  [unwired: 2 in, 2 out]
          }
          frame "Analog Out", "Motor", "PWM" {
            w257 = FALSE ("Visible")
            n143 = case shown="\"Analog Out\"" w256 {
              tunnel: [1.0 ("Value") -1.0 ("Value") 0.0 ("Value")] -> w255
              tunnel: [255.0 ("Value") 1.0 ("Value") 5.0 ("Value")] -> w254
              tunnel: [128.0 ("Value") 0.0 ("Value") 0.0 ("Value")] -> w253
              tunnel: [64.0 ("Value") 0.5 ("Value") 1.0 ("Value")] -> w252
              frame "PWM" {
              }
              frame "Motor", Default {
              }
              frame "Analog Out" {
              }
            }
            n144 = property on="Motor" class="Clust (strict)"("Visible"=TRUE) -> ()  [unwired: 2 in, 2 out]
            n145 = property on="Value" class="Slide (strict)"("Value"=w253, "Scale.Minimum"=w255, "Scale.Maximum"=w254, "Scale.Increment"=w252) -> ()  [unwired: 2 in, 2 out]
            n146 = property on="On/Off" class="Bool (strict)"("Visible"=w257) -> ()  [unwired: 2 in, 2 out]
            n147 = property on="Test Slider" class="Slide (strict)"("Visible"=w257) -> ()  [unwired: 2 in, 2 out]
            n148 = property on="Test Ring" class="Ring (strict)"("Visible"=w257) -> ()  [unwired: 2 in, 2 out]
            n149 = property on="Rev/Fwd" class="Clust (strict)"("Visible"=w257) -> ()  [unwired: 2 in, 2 out]
          }
          frame "Servo" {
            w273 = FALSE ("Visible")
            n150 = call <vilib>:"NT Read Number.vi"("Name"=w275) -> ("Numeric"=w274:dbl)  [unwired: 9 in, 1 out]
            n151 = property on="Test Slider" class="Slide (strict)"("Visible"=TRUE, "Scale.Maximum"=170.0 ("Scale.Range:Maximum")) -> ()  [unwired: 2 in, 2 out]
            n152 = local write "Test Slider"(w274) -> ()
            n153 = property on="Motor" class="Clust (strict)"("Visible"=w273) -> ()  [unwired: 2 in, 2 out]
            n154 = property on="Rev/Fwd" class="Clust (strict)"("Visible"=w273) -> ()  [unwired: 2 in, 2 out]
            n155 = property on="On/Off" class="Bool (strict)"("Visible"=w273) -> ()  [unwired: 2 in, 2 out]
            n156 = property on="Test Ring" class="Ring (strict)"("Visible"=w273) -> ()  [unwired: 2 in, 2 out]
          }
          frame "Relay", "Solenoid" {
            w276 = FALSE ("Visible")
            n157 = property on="Motor" class="Clust (strict)"("Visible"=w276) -> ()  [unwired: 2 in, 2 out]
            n158 = property on="Test Slider" class="Slide (strict)"("Visible"=w276) -> ()  [unwired: 2 in, 2 out]
            n159 = Search and Replace String(input string=w277, search string="/Value  **", replace string="/Direction") -> (result string=w283:string)  [unwired: 5 in, 3 out]
            n160 = property on="Test Ring" class="Ring (strict)"("Visible"=w276) -> ()  [unwired: 2 in, 2 out]
            n161 = call <vilib>:"NT Read String.vi"("Name"=w283) -> ("String"=w281:string)  [unwired: 9 in, 1 out]
            n162 = Equal?(x="Both directions", y=w281) -> (x = y?=w279:bool)
            n163 = Not(x=w279) -> (.not. x?=w280:bool)
            n164 = property on="Rev/Fwd" class="Clust (strict)"("Visible"=w279) -> ()  [unwired: 2 in, 2 out]
            n165 = property on="On/Off" class="Bool (strict)"("Visible"=w280, "Caption.Text"=w278) -> ()  [unwired: 2 in, 2 out]
          }
          frame "Compressor", "Digital Out" {
            w286 = FALSE ("Visible")
            # "Get direction and finish"
            n166 = property on="Motor" class="Clust (strict)"("Visible"=w286) -> ()  [unwired: 2 in, 2 out]
            n167 = property on="Test Slider" class="Slide (strict)"("Visible"=w286) -> ()  [unwired: 2 in, 2 out]
            n168 = property on="Test Ring" class="Ring (strict)"("Visible"=w286) -> ()  [unwired: 2 in, 2 out]
            n169 = property on="On/Off" class="Bool (strict)"("Visible"=TRUE, "Caption.Text"=w287) -> ()  [unwired: 2 in, 2 out]
            n170 = property on="Rev/Fwd" class="Clust (strict)"("Visible"=FALSE) -> ()  [unwired: 2 in, 2 out]
          }
          frame "Camera" {
            n171 = call <vilib>:"Get Last Path Segment.vi"("String in"=w294) -> ("String out"=w295:string)  [unwired: 10 in]
            n172 = property on="On/Off" class="Bool (strict)"("Visible"=FALSE) -> ()  [unwired: 2 in, 2 out]
            n173 = property on="Motor" class="Clust (strict)"("Visible"=FALSE) -> ()  [unwired: 2 in, 2 out]
            n174 = property on="Rev/Fwd" class="Clust (strict)"("Visible"=FALSE) -> ()  [unwired: 2 in, 2 out]
            n175 = case shown="\"White Balance  **\"" w295 {
              tunnel: w294 -> [w301 w310 w319 w328 w337 _ w343]
              tunnel: w293 -> [w299 w307 w316 w325 w334 _ _]
              frame "Size  **" {
                n176 = Index Array(array=w299) -> (element=w298:cluster{string[]})  [unwired: 1 in]
                n177 = call <vilib>:"NT Read String.vi"("Name"=w301) -> ("String"=w300:string)  [unwired: 9 in, 1 out]
                n178 = Unbundle(w298) -> (w296:string[])
                n179 = Match First String(2:w296, 3:w300) -> (0:w297:i32)  [unwired: 1 out]
                n180 = property on="Test Ring" class="Ring (strict)"("Value"=w297, "Strings []"=w296) -> ()  [unwired: 2 in, 2 out]
                n181 = property on="Test Ring" class="Ring (strict)"("Visible"=TRUE) -> ()  [unwired: 2 in, 2 out]
                n182 = property on="Test Slider" class="Slide (strict)"("Visible"=FALSE) -> ()  [unwired: 2 in, 2 out]
              }
              frame "White Balance  **" {
                n183 = Index Array(array=w307, index=1) -> (element=w308:cluster{string[]})
                n184 = call <vilib>:"NT Read String.vi"("Name"=w310) -> ("String"=w309:string)  [unwired: 9 in, 1 out]
                n185 = Unbundle(w308) -> (w305:string[])
                n186 = Match First String(2:w305, 3:w309) -> (0:w304:i32)  [unwired: 1 out]
                n187 = property on="Test Ring" class="Ring (strict)"("Value"=w304, "Strings []"=w305) -> ()  [unwired: 2 in, 2 out]
                n188 = property on="Test Ring" class="Ring (strict)"("Visible"=TRUE) -> ()  [unwired: 2 in, 2 out]
                n189 = property on="Test Slider" class="Slide (strict)"("Visible"=FALSE) -> ()  [unwired: 2 in, 2 out]
              }
              frame "Exposure  **" {
                n190 = Index Array(array=w316, index=2) -> (element=w317:cluster{string[]})
                n191 = call <vilib>:"NT Read String.vi"("Name"=w319) -> ("String"=w318:string)  [unwired: 9 in, 1 out]
                n192 = Unbundle(w317) -> (w313:string[])
                n193 = Match First String(2:w313, 3:w318) -> (0:w314:i32)  [unwired: 1 out]
                n194 = property on="Test Ring" class="Ring (strict)"("Value"=w314, "Strings []"=w313) -> ()  [unwired: 2 in, 2 out]
                n195 = property on="Test Ring" class="Ring (strict)"("Visible"=TRUE) -> ()  [unwired: 2 in, 2 out]
                n196 = property on="Test Slider" class="Slide (strict)"("Visible"=FALSE) -> ()  [unwired: 2 in, 2 out]
              }
              frame "Exposure Priority  **" {
                n197 = Index Array(array=w325, index=3) -> (element=w326:cluster{string[]})
                n198 = call <vilib>:"NT Read String.vi"("Name"=w328) -> ("String"=w327:string)  [unwired: 9 in, 1 out]
                n199 = Unbundle(w326) -> (w322:string[])
                n200 = Match First String(2:w322, 3:w327) -> (0:w323:i32)  [unwired: 1 out]
                n201 = property on="Test Ring" class="Ring (strict)"("Value"=w323, "Strings []"=w322) -> ()  [unwired: 2 in, 2 out]
                n202 = property on="Test Ring" class="Ring (strict)"("Visible"=TRUE) -> ()  [unwired: 2 in, 2 out]
                n203 = property on="Test Slider" class="Slide (strict)"("Visible"=FALSE) -> ()  [unwired: 2 in, 2 out]
              }
              frame "Color Enable  **" {
                n204 = Index Array(array=w334, index=4) -> (element=w335:cluster{string[]})
                n205 = call <vilib>:"NT Read String.vi"("Name"=w337) -> ("String"=w336:string)  [unwired: 9 in, 1 out]
                n206 = Unbundle(w335) -> (w331:string[])
                n207 = Match First String(2:w331, 3:w336) -> (0:w332:i32)  [unwired: 1 out]
                n208 = property on="Test Ring" class="Ring (strict)"("Value"=w332, "Strings []"=w331) -> ()  [unwired: 2 in, 2 out]
                n209 = property on="Test Ring" class="Ring (strict)"("Visible"=TRUE) -> ()  [unwired: 2 in, 2 out]
                n210 = property on="Test Slider" class="Slide (strict)"("Visible"=FALSE) -> ()  [unwired: 2 in, 2 out]
              }
              frame Default {
                n211 = property on="Test Ring" class="Ring (strict)"("Visible"=FALSE) -> ()  [unwired: 2 in, 2 out]
                n212 = property on="Test Slider" class="Slide (strict)"("Visible"=FALSE) -> ()  [unwired: 2 in, 2 out]
              }
              frame "Brightness  **", "Color Level  **", "Compression  **", "FPS  **", "Sharpness  **" {
                n213 = call <vilib>:"NT Read Number.vi"("Name"=w343) -> ("Numeric"=w342:dbl)  [unwired: 9 in, 1 out]
                n214 = local write "Test Slider"(w342) -> ()
                n215 = property on="Test Slider" class="Slide (strict)"("Visible"=TRUE, "Scale.Maximum"=100.0 ("Scale.Range:Maximum")) -> ()  [unwired: 2 in, 2 out]
                n216 = property on="Test Ring" class="Ring (strict)"("Visible"=FALSE) -> ()  [unwired: 2 in, 2 out]
              }
            }
          }
        }
        n217 = property on="Progress" class="Clust (strict)"("Visible"=FALSE) -> ()  [unwired: 2 in, 2 out]
      }
      event "Test Name": Mouse Enter {
        # "Populate the ring with the list of tests"
        n218 = event-data() -> ()  [unwired: 1 in, 1 out]
        n219 = call <vilib>:"NT Read String Array.vi"("Name"="TestMode/TestList") -> ("String Array"=w351:string[])  [unwired: 9 in, 1 out]
        n220 = Build Array (concatenate)("Select the test to run...", w351) -> (w350:string[])
        n221 = property on="Test Name" class="Ring (strict)"("Strings []"=w350) -> ()  [unwired: 2 in, 2 out]
      }
      event "Test Name": Value Change {
        w353 = FALSE ("Visible")
        # "Tell the robot the test name to run"
        n222 = event-data() -> ("NewVal"=w357:u16)  [unwired: 1 in]
        n223 = property on="Test Name" class="Ring (strict)"() -> ("Strings []"=w358:string[])  [unwired: 2 in, 2 out]
        n224 = local write "Progress"(T7 {"Test Progress"=0, "Test Progress Text"=""} ("Progress")) -> ()
        n225 = Index Array(array=w358, index=w357) -> (element=w356:string)
        n226 = call <vilib>:"NT Write String.vi"("String"=w356, "Name"="TestMode/TestName") -> ()  [unwired: 9 in, 1 out]
        n227 = property on="Progress" class="Clust (strict)"("Visible"=TRUE) -> ()  [unwired: 2 in, 2 out]
        n228 = property on="Motor" class="Clust (strict)"("Visible"=w353) -> ()  [unwired: 2 in, 2 out]
        n229 = property on="Test Slider" class="Slide (strict)"("Visible"=w353) -> ()  [unwired: 2 in, 2 out]
        n230 = property on="On/Off" class="Bool (strict)"("Visible"=w353) -> ()  [unwired: 2 in, 2 out]
        n231 = property on="Rev/Fwd" class="Clust (strict)"("Visible"=w353) -> ()  [unwired: 2 in, 2 out]
        n232 = property on="Test Ring" class="Ring (strict)"("Visible"=w353) -> ()  [unwired: 2 in, 2 out]
      }
      event "Select Auto": Mouse Enter {
        # "Populate the combo box with the list of autonomous options"
        n233 = event-data() -> ()  [unwired: 1 in, 1 out]
        n234 = call <vilib>:"NT Read String Array.vi"("Name"="Auto List") -> ("String Array"=w360:string[])  [unwired: 9 in, 1 out]
        n235 = property on="Select Auto" class="CmbBox"("Strings[]"=w360) -> ()  [unwired: 2 in, 2 out]
      }
      event "Select Auto": Value Change {
        # "User modified the Auto Selection. Write to NT variable so robot knows."
        n236 = event-data() -> ("NewVal"=w363:string)  [unwired: 1 in]
        n237 = call <vilib>:"NT Write String.vi"("String"=w363, "Name"="Auto Selector") -> ()  [unwired: 9 in, 1 out]
      }
      event "Command Selection": Value Change {
        # "Get the params and show in table"
        n238 = event-data() -> ("NewVal"=w369:i32)  [unwired: 1 in]
        n239 = property on="Command Selection" class="MCListbox (strict)"() -> ("ItemNames"=w367:string[][])  [unwired: 2 in, 2 out]
        n240 = call <vilib>:"WPI_DashboardUpdate Command Params.vi"("NewVal"=w369, "Commands"=w367, "Param Tbl"=w368) -> ()  [unwired: 8 in, 1 out]
      }
      event "Execute Command": Value Change {
        # "Started one, Unique ID holds\nresponse"
        n241 = event-data() -> ()  [unwired: 1 in, 1 out]
        n242 = property on="Command Selection" class="MCListbox (strict)"() -> ("ItemNames"=w380:string[][])  [unwired: 2 in, 2 out]
        n243 = Index Array(array=w380, index (row)="Command Selection", index (col)=0) -> (element=w378:string)
        n244 = call <vilib>:"Invoke Commands.vi"("Command Params"="Command Params", "Function Name"=w378) -> ("Params"=w374:u8, "Started"=w373:bool)  [unwired: 7 in, 1 out]
        n245 = Array Subset(array="Command Params", length (row)=w374) -> (w375:string[][])  [unwired: 3 in]
        n246 = Select(t="Executing" ("Cmd Status"), s=w373, f="" ("Cmd Status")) -> (s? t:f=→"Cmd Status":string)
      }
      event "Command Selection": Double Click {
        n247 = event-data() -> ("Row"=w388:i32)  [unwired: 1 in]
        n248 = property on="Command Selection" class="MCListbox (strict)"() -> ("ItemNames"=w391:string[][])  [unwired: 2 in, 2 out]
        n249 = local read "Command Params"() -> (w387:string[][])
        n250 = Index Array(array=w391, index (row)=w388, index (col)=0) -> (element=w389:string)
        n251 = call <vilib>:"Invoke Commands.vi"("Command Params"=w387, "Function Name"=w389) -> ("Params"=w386:u8, "Started"=w381:bool)  [unwired: 7 in, 1 out]
        n252 = Array Subset(array=w387, length (row)=w386) -> (w385:string[][])  [unwired: 3 in]
        n253 = Select(t="Executing" ("Cmd Status"), s=w381, f="" ("Cmd Status")) -> (s? t:f=w382:string)
        n254 = local write "Cmd Status"(w382) -> ()
      }
      event "CheckList": Double Click {
        # "Shift clears all"
        # "Update symbols on the listbox"
        n255 = event-data() -> ("PlatMods.Shift"=w393:bool, "Row"=w395:i32)  [unwired: 1 in]
        n256 = case shown="True" w393 {
          tunnel: w395 -> [w399 _]
          tunnel: 1 -> [w398 _]
          frame False {
            n257 = property on="CheckList" class="LstBox (strict)"() -> ("Item Symbols"=w397:i32[])  [unwired: 2 in, 2 out]
            n258 = Replace Array Subset(array=w397, new element=w398, index=w399) -> (w396:i32[])
            n259 = property on="CheckList" class="LstBox (strict)"("Item Symbols"=w396) -> ()  [unwired: 2 in, 2 out]
          }
          frame True {
            w400 = 0 ("Top Row")
            n260 = property on="CheckList" class="LstBox (strict)"() -> ("Number of Rows"=w402:u32)  [unwired: 2 in, 2 out]
            n261 = Initialize Array(0, w402) -> (w401:i32[])
            n262 = property on="CheckList" class="LstBox (strict)"("Top Row"=w400, "Value"=w400, "Item Symbols"=w401) -> ()  [unwired: 2 in, 2 out]
          }
        }
      }
      event "CheckList": Key Down {
        # "Update symbols on the listbox\nLeft and right keys check and uncheck"
        n263 = event-data() -> ("VKey"=w406:T24)  [unwired: 1 in]
        n264 = case shown="\"Left\", \"Right\"" w406 {
          selector: w406 -> [w411 _]
          tunnel: eventvkey."Left" ("VKey") -> [w409 _]
          frame "Left", "Right" {
            n265 = Equal?(x=w409, y=w411) -> (x = y?=w410:bool)
            n266 = Select(t=0, s=w410, f=1) -> (s? t:f=w412:i32)
            n267 = property on="CheckList" class="LstBox (strict)"() -> ("Item Symbols"=w415:i32[])  [unwired: 2 in, 2 out]
            n268 = Replace Array Subset(array=w415, new element=w412, index="CheckList") -> (w414:i32[])
            n269 = property on="CheckList" class="LstBox (strict)"("Item Symbols"=w414) -> ()  [unwired: 2 in, 2 out]
          }
          frame Default {
          }
        }
      }
      event "Motor.Enable": Value Change {
        # "When the test mode otor enable helper is set, update that\ntree row item's value"
        n270 = event-data() -> ("NewVal"=w421:bool)  [unwired: 1 in]
        n271 = Unbundle("Motor") -> ("Value"=w420:dbl)  [unwired: 1 out]
        n272 = Select(t=w420, s=w421, f=0.0) -> (s? t:f=w418:dbl)
        n273 = call <vilib>:"NT Write Number.vi"("Numeric"=w418, "Name"=w417) -> ()  [unwired: 9 in, 1 out]
      }
      event "Test Slider": Value Change {
        # "When the test mode slider helper is set, update that\ntree row item's value"
        n274 = event-data() -> ("NewVal"=w424:dbl)  [unwired: 1 in]
        n275 = call <vilib>:"NT Write Number.vi"("Numeric"=w424, "Name"=w425) -> ()  [unwired: 9 in, 1 out]
      }
      event "On/Off": Value Change {
        # "When the test mode on/off helper value is set, update that\ntree row item's value"
        n276 = event-data() -> ("NewVal"=w429:bool)  [unwired: 1 in]
        n277 = Boolean To (0,1)(Boolean=w429) -> (0, 1=w428:i16)
        n278 = call <vilib>:"NT Write Number.vi"("Numeric"=w428, "Name"=w427) -> ()  [unwired: 9 in, 1 out]
      }
      event "Rev/Fwd": Value Change {
        # "When the test mode helper value for relays is set, update that\ntree row item's value"
        n279 = event-data() -> ("NewVal.Forward"=w437:bool, "NewVal.Reverse"=w436:bool)  [unwired: 1 in]
        n280 = Boolean To (0,1)(Boolean=w437) -> (0, 1=w433:i16)
        n281 = Boolean To (0,1)(Boolean=w436) -> (0, 1=w435:i16)
        n282 = Negate(x=w435) -> (-x=w434:i16)
        n283 = Add(x=w433, y=w434) -> (x+y=w432:i16)
        n284 = call <vilib>:"NT Write Number.vi"("Numeric"=w432, "Name"=w431) -> ()  [unwired: 9 in, 1 out]
      }
      event "Test Ring": Value Change {
        # "When a test mode helper value is selected from the ring,\nset the tree item's variable to the string value"
        n285 = event-data() -> ("NewVal"=w441:u16)  [unwired: 1 in]
        n286 = property on="Test Ring" class="Ring (strict)"() -> ("Strings []"=w442:string[])  [unwired: 2 in, 2 out]
        n287 = Index Array(array=w442, index=w441) -> (element=w440:string)
        n288 = call <vilib>:"NT Write String.vi"("String"=w440, "Name"=w439) -> ()  [unwired: 9 in, 1 out]
      }
      event "Rec Mode": Value Change {
        # "Update globals for recording mode and path to read log from.\nClear when logging and let NetworkTables set path for vision to\nuse."
        n289 = event-data() -> ("NewVal"=w453:enum32{"Stop", "Record", "Playback"})  [unwired: 1 in]
        n290 = global write "WPI_DashboardLogging Global.vi" "Logging Filename"(path "") -> ()
        n291 = global write "WPI_DashboardLogging Global.vi" "Recording"(w453) -> ()
        n292 = case shown="\"Playback\"" w453 {
          tunnel: w452 -> [_ w455 w464]
          tunnel: [_ _ w463] -> w450
          tunnel: [_ _ w462] -> _
          tunnel: w448 -> [_ _ w460]
          tunnel: cluster{i32, i32} {-250, 170} -> [_ _ w459]
          tunnel: [_ _ T25 {"Image Size"=TRUE, "Image Type"=TRUE, "Pixel Value"=TRUE, "ROI Information"=TRUE, "Zoom Factor"=FALSE} ("Image Information Shown:All Elements")] -> w443
          tunnel: [_ _ TRUE ("Zoom Factor")] -> w444
          tunnel: w446 -> [_ _ w456]
          frame Default {
          }
          frame "Stop", "Record" {
            # "Place Window too"
            n293 = invoke class="VI" method="FP.Close"(reference=w455) -> (reference out=w454:refnum<vi>)  [unwired: 2 in, 2 out]
            n294 = invoke class="VI" method="Abort VI"(reference=w454) -> ()  [unwired: 2 in, 3 out]
          }
          frame "Playback" {
            n295 = call "Open Playback Panel.vi"("Offset"=w459, "DB VI Ref"=w460, "Playback in"=w464) -> ("Playback out"=w461:refnum<vi>)  [unwired: 8 in]
            n296 = register-events(w461, w456) -> (reference out=w463:refnum<event-registration>, error out=w462:errorcluster)  [unwired: 2 in]
          }
        }
        n297 = property on="Camera Image Right" class="ImageControl"("Image Information Shown"=w443, "Image Information Visible"=w444) -> ()  [unwired: 2 in, 2 out]
        n298 = property on="Camera Image" class="ImageControl"("Image Information Shown"=w443, "Image Information Visible"=w444) -> ()  [unwired: 2 in, 2 out]
        n299 = call <vilib>:"WPI_DashboardNT Log FieldName Cache.vi"("Operation"=enum16{"Lookup/Add", "Index", "Clear"}."Clear") -> ()  [unwired: 8 in, 3 out]
      }
      event Panel Close {
        w466 = enum32{"Stop", "Record", "Playback"}."Stop" ("Rec Mode")
        # "Playback window has been closed, abort"
        n300 = event-data() -> ()  [unwired: 1 in, 4 out]
        n301 = local write "Rec Mode"(w466) -> ()
        n302 = global write "WPI_DashboardLogging Global.vi" "Recording"(w466) -> ()
      }
      event Panel Close {
        # "Abort playback window and ourself"
        n303 = event-data() -> ()  [unwired: 1 in, 4 out]
        n304 = invoke class="VI" method="FP.Close"(reference=w470) -> (reference out=w469:refnum<vi>)  [unwired: 2 in, 2 out]
        n305 = invoke class="VI" method="Abort VI"(reference=w469) -> (error out=w468:errorcluster)  [unwired: 2 in, 2 out]
        n306 = invoke class="VI" method="Abort VI"(error in=w468) -> ()  [unwired: 2 in, 3 out]
      }
      event User Event {
        n307 = event-data() -> ("IDs"=w477:cluster{"RPC field ID":u16, "Unique ID":u16}, "String"=w476:string)  [unwired: 1 in]
        n308 = Bundle("IDs"=w477, "String"=w476) -> (w475:T10)  [unwired: 1 in]
        n309 = call <vilib>:"Retrieve RPC Response.vi"("RPC Response"=w475) -> ("Output"=w473:string[][])  [unwired: 10 in]
        n310 = Build Array (concatenate)(w471, w473) -> (w472:string[][])
        n311 = local write "Command Params"(w472) -> ()
        n312 = local write "Cmd Status"("" ("Cmd Status")) -> ()
      }
      event "Tree": Double Click {
        n313 = event-data() -> ("PlatMods"=w483:T28, "Tag"=w480:string)  [unwired: 1 in]
        n314 = Unbundle(w483) -> ("Shift"=w482:bool)  [unwired: 4 out]
        n315 = String Subset(string=w480, length (rest)=1 ("length (rest)")) -> (substring=w479:string)  [unwired: 1 in]
        n316 = Not(x=w482) -> (.not. x?=w481:bool)
        n317 = case shown="\"/\"" w479 {
          tunnel: w480 -> [_ w486]
          tunnel: w481 -> [_ w485]
          frame Default {
          }
          frame "/" {
            n318 = call <vilib>:"NT Update Persistence.vi"("Persistence"=w485, "Name"=w486) -> ()  [unwired: 9 in, 1 out]
          }
        }
      }
    }
  }
  n319 = while {
    tunnel: w66 -> [w488]
    i -> [w491]
    stop <- FALSE stop-if-true
    n320 = Wait (ms)(milliseconds to wait=u32 100) -> ()  [unwired: 1 out]
    n321 = case shown="\"Playback\"" "Rec Mode" {
      tunnel: w491 -> [_ _ w506]
      tunnel: [u32 2829099 ("Base Color") u32 11141120 ("Target Color") w495] -> w487
      frame "Stop", Default {
        # "Reset the color, extra updates don't cost much"
      }
      frame "Record" {
      }
      frame "Playback" {
        # "Playback"
        n322 = Quotient & Remainder(x=w506, y=u32 50 ("milliseconds to wait")) -> (x-y*floor(x/y)=w502:u32)  [unwired: 1 out]
        n323 = Divide(x=w502, y=u32 50 ("milliseconds to wait")) -> (x/y=w499:dbl)
        n324 = Multiply(x=6.283185307179586, y=w499) -> (x*y=w504:dbl)
        n325 = Sine(x=w504) -> (sin(x)=w503:dbl)
        n326 = Absolute Value(x=w503) -> (abs(x)=w496:dbl)
        n327 = call "Interpolate RGB Color.vi"("Proportion"=w496, "Target Color"=u32 30976, "Base Color"=u32 2829099) -> ("Result Color"=w495:u32)  [unwired: 8 in]
      }
    }
    n328 = property class="Pane"(reference=w488, "PaneColor"=w487) -> ()  [unwired: 1 in, 2 out]
  }
  n329 = local write "Dashboard Tab"(T3."Drive" ("Dashboard Tab")) -> ()
  n330 = property on="On/Off" class="Bool (strict)"("Visible"=w37) -> ()  [unwired: 2 in, 2 out]
  n331 = property on="Motor" class="Clust (strict)"("Visible"=w37) -> ()  [unwired: 2 in, 2 out]
  n332 = property on="Progress" class="Clust (strict)"("Visible"=w37) -> ()  [unwired: 2 in, 2 out]
  n333 = property on="Test Ring" class="Ring (strict)"("Visible"=w37) -> ()  [unwired: 2 in, 2 out]
  n334 = property on="Rev/Fwd" class="Clust (strict)"("Visible"=w37) -> ()  [unwired: 2 in, 2 out]
  n335 = while {
    tunnel: u16 1741 ("timeout ms (25000)") -> [w508]
    stop <- FALSE stop-if-true
    n336 = TCP Create Listener(10:w508) -> (0:w507:errorcluster, 3:w509:refnum<k5>)  [unwired: 4 in, 1 out]
    n337 = case shown="No Error" w507 {
      selector: w507 -> [w511 _]
      tunnel: w509 -> [w512 _]
      frame No Error {
        n338 = while {
          tunnel: w512 -> [w515]
          tunnel: w511 -> [w514]
          stop <- FALSE stop-if-true
          n339 = TCP Wait On Listener(8:w514, 11:w515) -> (0:w516:errorcluster, 4:w517:refnum<k5>)  [unwired: 2 in, 3 out]
          n340 = local write "TCP"(w517) -> ()
          n341 = case shown="No Error" w516 {
            frame No Error {
            }
            frame Error {
              n342 = Wait (ms)(milliseconds to wait=u32 1000) -> ()  [unwired: 1 out]
            }
          }
        }
      }
      frame Error {
        n343 = Wait (ms)(milliseconds to wait=u32 1000) -> ()  [unwired: 1 out]
      }
    }
  }
  n344 = local write "Command Selection"(u16 0 ("milliseconds to wait")) -> ()
  n345 = local write "Command Params"(string[][] [] ("Command Params")) -> ()
  n346 = global write "WPI_DashboardLogging Global.vi" "Recording"(w60) -> ()
  n347 = local write "Rec Mode"(w60) -> ()
  n348 = call <vilib>:"NT Write String.vi"("String"="Select Auto", "Name"="Auto Selector") -> ()  [unwired: 9 in, 1 out]
